vi "create data file.vi"(2 "create file":bool=TRUE, 7 "exp exec in":T1={"data file"={"autosave"=FALSE, "File refnum"=refnum, "data file path"=path ""}, "T log file"={"File refnum"=refnum, "T log file path"=path "", "exists"=FALSE}, "exp seq"={"wave params"={"Num of avg"=0, "Num points"=1000, "Meas rate (Hz)"=100000.0}, "Setpoints"=[], "#"=-1, "index"=-1, "elapsed time (s)"=0.0, "set time (s)"=0.0, "min settle (s)"=30.0, " Exec Status"=enum."Settling"}, "error"={"status"=FALSE, "code"=0, "source"=""}}, 13 "Header":string="This is a C(T) experiment being done in Physics 3600.\nIt records the decay response of an RC circuit where the capacitance is a strong function of temperature." caption="Header Comments", 14 "autosave":bool caption="autosave when complete") -> (8 "exp exec out":T1={"data file"={"autosave"=FALSE, "File refnum"=refnum, "data file path"=path "C:/Users/Paul Dixon/work/Teaching/P3600 F20/P3600 F20 instr/Development/play/bug C(T) sequence/full bug C(T) exp/saved data/bug data 11 20 2020 4 34 52 PM.txt"}, "T log file"={"File refnum"=refnum, "T log file path"=path "", "exists"=FALSE}, "exp seq"={"wave params"={"Num of avg"=0, "Num points"=1000, "Meas rate (Hz)"=100000.0}, "Setpoints"=[], "#"=-1, "index"=-1, "elapsed time (s)"=0.0, "set time (s)"=0.0, "min settle (s)"=30.0, " Exec Status"=enum."Settling"}, "error"={"status"=FALSE, "code"=0, "source"=""}}, 15 "full \nheader":string="This is a C(T) experiment being done in Physics 3600.\nIt records the decay response of an RC circuit where the capacitance is a strong function of temperature.\n\n11/20/2020\n4:34 PM\n\nwaveform params\tn meas\tindex\ttime (S)\ttemp (C)\tcapacitance (F)\tnormalized waveforms\n\n<data below>\n")   [LabVIEW 2019]
doc: "This is a Bug C(T) subVI.\n\nThis subVI creates the data file for the bug experiment and saves the header data.\nThe data is apppended at the end of the experiment.\n\nPaul K Dixon\nP3600\nCSUSB Physics"
uses:
  typedefs/PID exec cluster.ctl
  typedefs/data file info.ctl
  typedefs/bug temp file info.ctl
  typedefs/exp seq cluster.ctl
  typedefs/wvfm acq params.ctl
  typedefs/bug meas status.ctl
panel:
  out "exists":bool=TRUE
  out "file refnum out":refnum<file>
  in  "String":string="waveform params\tn meas\tindex\ttemp (C)\ttime (S)\tcapacitance (F)\tnormalized waveforms"
  out "file path":path=path "C:/Users/Paul Dixon/work/Teaching/P3600 F20/P3600 F20 instr/Development/play/bug C(T) sequence/full bug C(T) exp/saved data/bug data 11 20 2020 4 34 52 PM.txt"
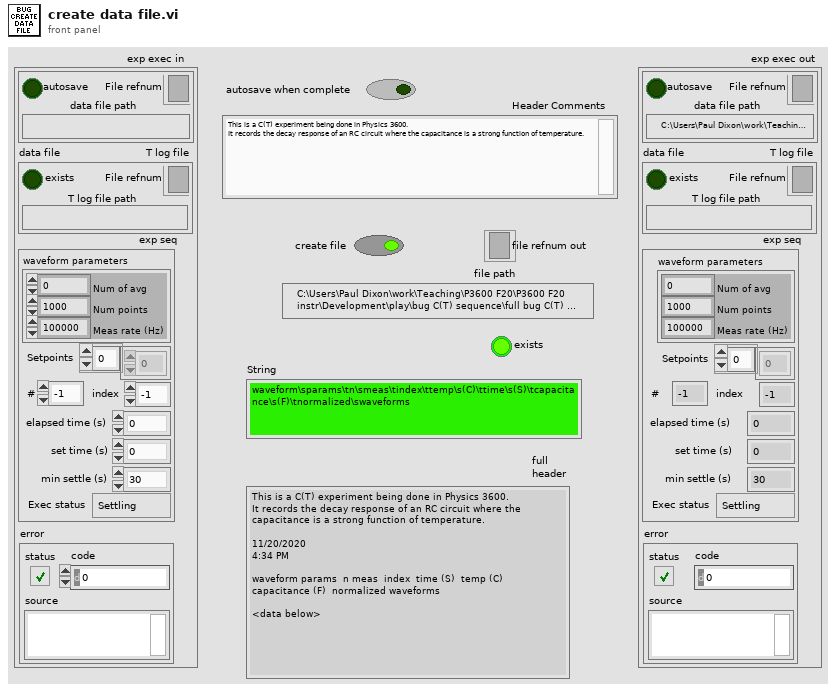
[diagram p1: front panel]
types:
  T1 = typedef "PID exec cluster.ctl" = cluster{"data file":T2, "T log file":T3, "exp seq":T4, "error":errorcluster}
  T2 = typedef "data file info.ctl" = cluster{"autosave":bool, "File refnum":refnum<file>, "data file path":path}
  T3 = typedef "bug temp file info.ctl" = cluster{"File refnum":refnum<file>, "T log file path":path, "exists":bool}
  T4 = typedef "exp seq cluster.ctl" = cluster{"wave params":T5, "Setpoints":dbl[], "#":i32, "index":i32, "elapsed time (s)":dbl, "set time (s)":dbl, "min settle (s)":dbl, " Exec Status":T6}
  T5 = typedef "wvfm acq params.ctl" = cluster{"Num of avg":i32, "Num points":i32, "Meas rate (Hz)":dbl}
  T6 = typedef "bug meas status.ctl" = enum32{"Settling", "Measuring", "Holding", "Exit"}
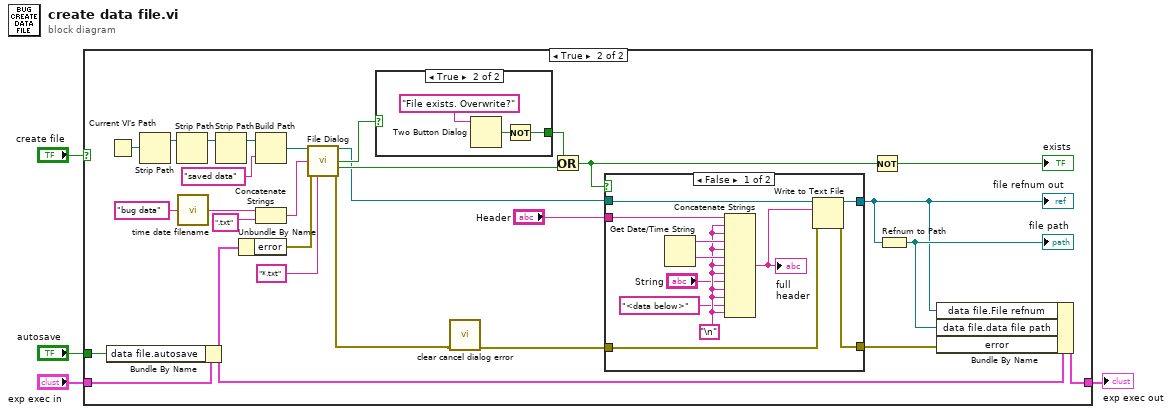
[diagram p0: block diagram]
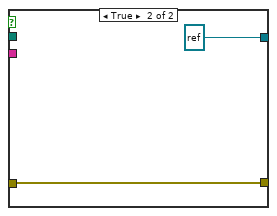
[diagram p3: hidden frame]
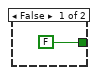
[diagram p4: hidden frame]
diagram:
  n1 = case shown="True" "create file" {
    tunnel: "exp exec in" -> [w5 w32]
    tunnel: [w5 w30] -> w4
    tunnel: "autosave" -> [_ w6]
    frame False {
    }
    frame True {
      n2 = Bundle By Name(cluster=w32, "data file.autosave"=w6) -> (w7:T1)
      n3 = Current VI's Path() -> (path=w24:path)
      n4 = Strip Path(path=w24) -> (stripped path=w25:path)  [unwired: 1 out]
      n5 = Strip Path(path=w25) -> (stripped path=w16:path)  [unwired: 1 out]
      n6 = call "time date filename.vi"("file name in"="bug data" ("name or relative path")) -> ("time date file name out"=w11:string)  [unwired: 14 in]
      n7 = Strip Path(path=w16) -> (stripped path=w15:path)  [unwired: 1 out]
      n8 = Unbundle By Name(w7) -> ("error"=w31:errorcluster)
      n9 = Build Path(base path=w15, name or relative path="saved data") -> (appended path=w13:path)
      n10 = Concatenate Strings(w11, ".txt" ("name or relative path")) -> (w9:string)
      n11 = call "File Dialog"("start path"=w13, "default name"=w9, "error in"=w31, "pattern (all files)"="*.txt") -> ("selected path"=w18:path, "exists"=w20:bool, "cancelled"=w19:bool, "error out"=w17:errorcluster)  [unwired: 8 in]
      n12 = case shown="True" w20 {
        tunnel: [FALSE ("T button?") w48] -> w23
        frame False {
        }
        frame True {
          n13 = Two Button Dialog(message="File exists. Overwrite?") -> (T button?=w49:bool)  [unwired: 2 out]
          n14 = Not(x=w49) -> (.not. x?=w48:bool)
        }
      }
      n15 = call "clear cancel dialog error.vi"("error in"=w17) -> ("error out"=w22:errorcluster)  [unwired: 14 out]
      n16 = Or(x=w23, y=w19) -> (x .or. y?=w33:bool)
      n17 = case shown="False" w33 {
        tunnel: "Header" -> [w37 _]
        tunnel: w18 -> [w43 _]
        tunnel: w22 -> [w42 w45]
        tunnel: [w41 w45] -> w29
        tunnel: [w40 refnum<file> refnum ("refnum out")] -> w27
        frame False {
          w36 = "\n"
          n18 = Get Date/Time String() -> (date string=w39:string, time string=w38:string)  [unwired: 3 in]
          n19 = Concatenate Strings(w37, w36, w36, w39, w36, w38, w36, w36, "String", w36, w36, "<data below>", w36) -> (w44:string)
          "full \nheader" <- w44
          n20 = Write to Text File(file (use dialog)=w43, text=w44, error in=w42) -> (refnum out=w40:refnum<file>, error out=w41:errorcluster)  [unwired: 2 out]
        }
        frame True {
        }
      }
      "file refnum out" <- w27
      n21 = Not(x=w33) -> (.not. x?=→"exists":bool)
      n22 = Refnum to Path(1:w27) -> (0:w28:path)
      "file path" <- w28
      n23 = Bundle By Name(cluster=w7, "data file.File refnum"=w27, "data file.data file path"=w28, "error"=w29) -> (w30:T1)
    }
  }
  "exp exec out" <- w4
